vi "AssetInterface_Write Process Name.vi"(10 "Process Name":string, 11 "AssetInterface in":refnum<class "AssetInterface.lvclass">) -> (3 "AssetInterface out":refnum<class "AssetInterface.lvclass">)   [LabVIEW 2015, in "AssetInterface.lvclass"]
uses:
  AssetInterface.lvclass
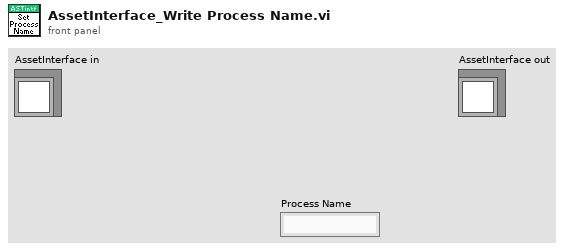
[diagram p1: front panel]
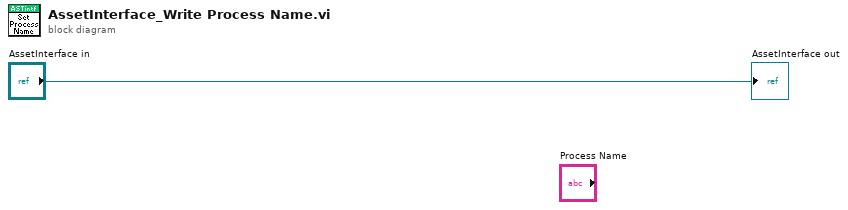
[diagram p0: block diagram]
diagram:
  "AssetInterface out" <- "AssetInterface in"
